vi "GPS Set Target Loop.vi"   [LabVIEW 2009]
uses:
  <vilib>/Platform/TimedLoop/XDataNode/XDataNode.xnode
  <vilib>/Platform/TimedLoop/XDataNode/loadlvalarms.vi
  <vilib>/Platform/TimedLoop/XDataNode/timing_clust.ctl
  <vilib>/Platform/TimedLoop/XDataNode/nitl_modes.ctl
  <vilib>/Platform/TimedLoop/XDataNode/wakeup.ctl
  TypeDefs/State Machine/Main State.ctl
  TypeDefs/Sensor TypeDefs/GPS Data.ctl
  Functional Global Variables/Actions for FG's.ctl
  <vilib>/Platform/TimedLoop/XDataNode/XDNodeRunTimeDep.lvlib
types:
  T1 = typedef "XDNodeRunTimeDep.lvlib/timing_clust.ctl" = cluster{"Expected End [f-1]":u64, "Actual End [f-1]":u64, "Finished Late? [f-1]":bool, "Expected End [i-1]":u64, "Actual End [i-1]":u64, "Finished Late? [i-1]":bool, "Expected Start [i]":u64, "Actual Start [i]":u64, "Expected Start [f]":u64, "Actual Start [f]":u64, "Source Name":string, "Structure Name":string, "Period":i64, "Deadline":i64, "Offset":i64, "Start":i64, "Priority":i32, "Timeout":i32, "Mode":T2, "Wakeup Reason":T3, "Error":errorcluster, "Source Type":string, "Secondary Source Type":string, "Global End Time":u64, "Global Start Time":u64, "Frame Duration":u64, "Iteration Duration":u64, "Assigned CPU":i32, "I/O Scan Engine Mode":u32}
  T2 = typedef "XDNodeRunTimeDep.lvlib/nitl_modes.ctl" = enum32{"No Change", "Process missed periods, maintain original phase", "Discard missed periods, maintain original phase", "Process missed periods, ignore original phase", "Discard missed periods, ignore original phase"}
  T3 = typedef "XDNodeRunTimeDep.lvlib/wakeup.ctl" = enum32{"Normal", "Aborted", "Asynchronous wakeup", "Timing source error", "Timed loop error", "Timeout"}
  T4 = typedef "Main State.ctl" = enum16{"Startup", "Wait for Init", "Initialize Sensors", "Wait for Saftey Disable", "Check Saftey", "Wait for GO", "Run", "Remote Control", "Stop"}
  T5 = typedef "Actions for FG's.ctl" = enum16{"Read", "Write"}
  T6 = typedef "GPS Data.ctl" = cluster{"Latitude":dbl, "Longitude":dbl}
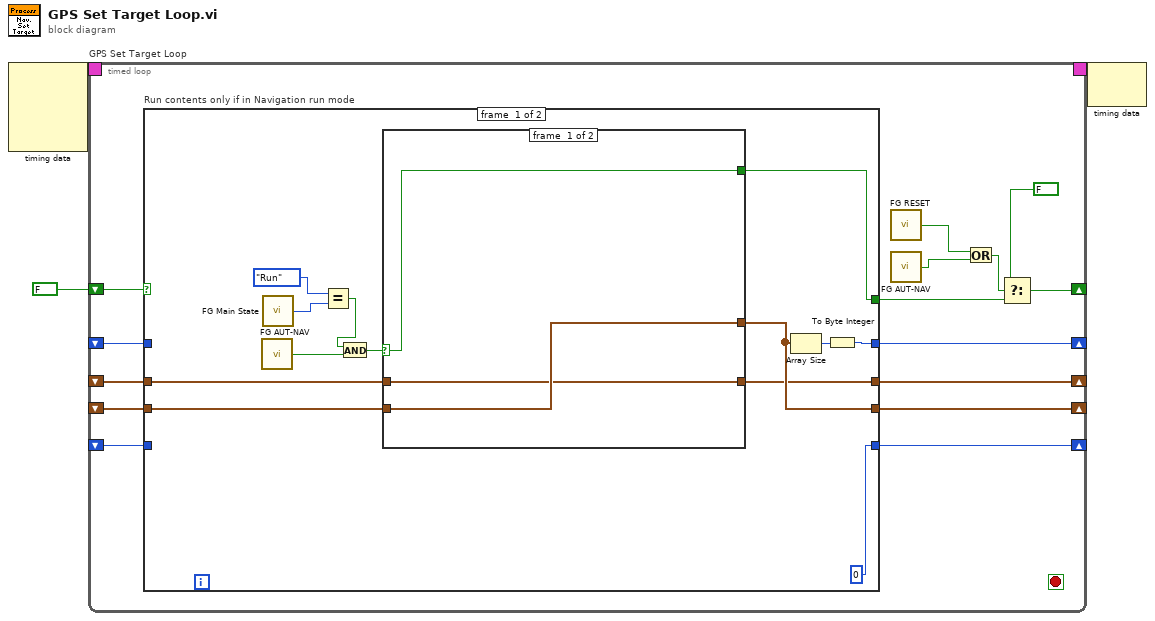
[diagram p0: block diagram]
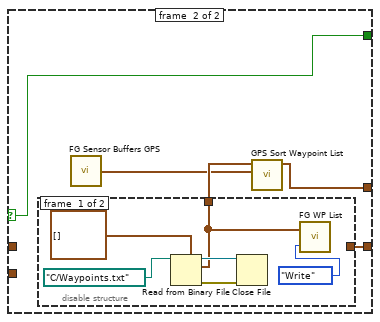
[diagram p2: hidden frame]
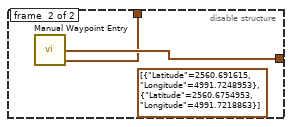
[diagram p3: hidden frame]
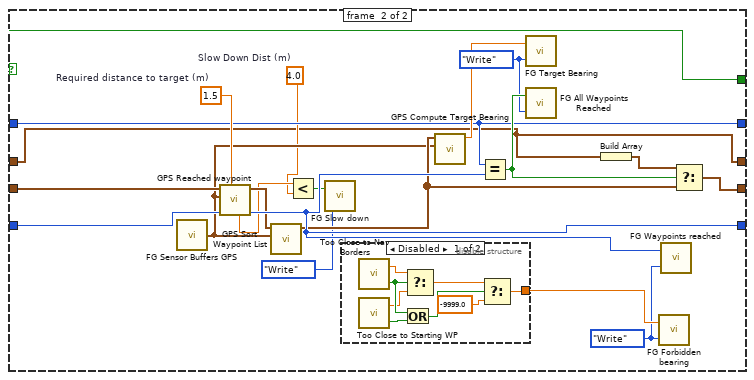
[diagram p4: hidden frame]
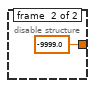
[diagram p5: hidden frame]
diagram:
  n1 = node-c288() -> (w3:T1)  [unwired: 4 in]
  n2 = timed-loop "GPS Set Target Loop" {
    timing: w3 -> [_]
    timing-out: [_] -> w2
    shift-right: [w16] -> _
    shift-left: _ -> [w18]
    shift-right: [w14] -> _
    shift-left: _ -> [w15]
    shift-right: [w10] -> _
    shift-left: FALSE ("t") -> [w9]
    shift-right: [w13] -> _
    shift-left: _ -> [w17]
    shift-right: [w8] -> _
    shift-left: _ -> [w7]
    stop <- _ stop-if-true
    n3 = case "Run contents only if in Navigation run mode" shown="False" w9 {
      selector: w9 -> [_ w57]
      tunnel: w18 -> [_ w67]
      tunnel: w17 -> [_ w56]
      tunnel: [i8 0 ("Number of WP Reached OUT") w66] -> w16
      tunnel: w15 -> [w24 w65]
      tunnel: [w22 w60] -> w14
      tunnel: [w27 w57] -> w11
      tunnel: [w25 w56] -> w13
      tunnel: [w21 w48] -> w8
      tunnel: w7 -> [w20 w48]
      frame #0 {
        n4 = call "FG AUT-NAV.vi"() -> ("Aut/!Nav out"=w19:bool)  [unwired: 2 in]
        n5 = call "FG Main State.vi"() -> ("Main State out"=w28:T4)  [unwired: 2 in]
        n6 = Equal?(x=Main_State."Run" ("Main State out"), y=w28) -> (x = y?=w30:bool)
        n7 = And(x=w30, y=w19) -> (x .and. y?=w31:bool)
        n8 = case shown="True" w31 {
          selector: w31 -> [w34 w39]
          tunnel: [w34 w39] -> w27
          tunnel: w24 -> [w33 _]
          tunnel: [w33 w36] -> w22
          tunnel: [w32 w35] -> w21
          tunnel: w20 -> [w32 _]
          frame #0 {
          }
          frame #1 {
            n9 = disable-structure shown="Enabled" {
              disable-tunnel: [w40 w46] -> w38
              disable-tunnel: [_ w47] -> w35
              frame #0 {
                n10 = Read from Binary File(5:T6[] [] ("Unsorted Waypoint List"), 11:path "C:/Waypoints.txt" ("file path (use dialog)")) -> (0:w44:errorcluster, 2:w40:T6[], 3:w43:refnum<file>)  [unwired: 4 in, 1 out]
                n11 = Close File(refnum=w43, error in=w44) -> ()  [unwired: 2 out]
                n12 = call "FG WP List.vi"("FG Action (Read)"=Actions_for_FG's."Write", "Sorted Waypoints in"=w40) -> ()  [unwired: 1 out]
              }
              frame #1 {
                (unwired) T6[] [{"Latitude"=2560.691615, "Longitude"=4991.7248953}, {"Latitude"=2560.6754953, "Longitude"=4991.7218863}] ("Unsorted Waypoint List")
                n13 = call "Manual Waypoint Entry.vi"() -> ("WP List Out"=w46:T6[], "Nav Course Ending Location"=w47:T6)  [unwired: 3 in, 1 out]
              }
            }
            n14 = call "FG Sensor Buffers GPS.vi"() -> ("GPS Buffer out"=w37:T6)  [unwired: 2 in]
            n15 = call "GPS Sort Waypoint List.vi"("Current co-ordinate"=w37, "Unsorted Waypoint List"=w38) -> ("Sorted Waypoints"=w36:T6[])  [unwired: 9 in]
          }
        }
        n16 = Array Size(array=w22) -> (size(s)=w26:i32)
        n17 = To Byte Integer(number=w26) -> (8bit integer=w25:i8)
      }
      frame #1 {
        w51 = 4.0  # Slow Down Dist (m)
        w58 = Actions_for_FG's."Write" ("FG Action (Read)")
        w63 = Actions_for_FG's."Write" ("FG Action (Read)")
        w62 = 1.5  # Required distance to target (m)
        n18 = call "FG Sensor Buffers GPS.vi"() -> ("GPS Buffer out"=w53:T6)  [unwired: 2 in]
        n19 = call "GPS Reached waypoint.vi"("Required distance to target (meters)"=w62, "Number of WP Reached IN"=w67, "Current Co-ordinates"=w53, "Waypoint List In"=w65) -> ("Number of WP Reached OUT"=w66:i8, "Waypoint List Out"=w55:T6[], "Distance to Target (meters)"=w52:dbl)  [unwired: 4 in, 1 out]
        n20 = call "GPS Sort Waypoint List.vi"("Current co-ordinate"=w53, "Unsorted Waypoint List"=w55) -> ("Sorted Waypoints"=w54:T6[])  [unwired: 9 in]
        n21 = Less?(x=w52, y=w51) -> (x < y?=w50:bool)
        n22 = call "FG Slow down.vi"("FG Action (Read)"=Actions_for_FG's."Write", "Slow down in"=w50) -> ()  [unwired: 1 out]
        n23 = disable-structure shown="Disabled" {
          disable-tunnel: [w69 -9999.0 ("Forbidden bearing in")] -> w64
          frame #0 {
            n24 = call "Too Close to Nav Borders.vi"() -> ("Too Close?"=w73:bool, "Bearing to Avoid"=w72:dbl)  [unwired: 2 in]
            n25 = call "Too Close to Starting WP.vi"() -> ("Too Close?"=w76:bool, "Bearing to Avoid"=w71:dbl)  [unwired: 2 in]
            n26 = Or(x=w73, y=w76) -> (x .or. y?=w75:bool)
            n27 = Select(t=w72, s=w73, f=w71) -> (s? t:f=w70:dbl)
            n28 = Select(t=w70, s=w75, f=-9999.0) -> (s? t:f=w69:dbl)
          }
          frame #1 {
          }
        }
        n29 = call "GPS Compute Target Bearing.vi"("Current co-ordinates"=w53, "GPS Waypoint List Out"=w54) -> ("Target Bearing (degrees)"=w68:dbl)  [unwired: 8 in]
        n30 = Equal?(x=w56, y=w66) -> (x = y?=w59:bool)
        n31 = call "FG Target Bearing.vi"("FG Action (Read)"=w58, "Target Bearing in"=w68) -> ()  [unwired: 1 out]
        n32 = call "FG All Waypoints Reached.vi"("FG Action (Read)"=w58, "All waypoints reached in"=w59) -> ()  [unwired: 1 in, 1 out]
        n33 = Build Array(w48) -> (w61:T6[])
        n34 = call "FG Forbidden bearing.vi"("FG Action (Read)"=w63, "Forbidden bearing in"=w64) -> ()  [unwired: 1 out]
        n35 = call "FG Waypoints reached.vi"("FG Action (Read)"=w63, "Waypoints reached in"=w66) -> ()  [unwired: 1 in, 1 out]
        n36 = Select(t=w61, s=w59, f=w54) -> (s? t:f=w60:T6[])
      }
    }
    n37 = call "FG RESET.vi"() -> ("RESET out"=w6:bool)  [unwired: 2 in]
    n38 = call "FG AUT-NAV.vi"() -> ("Aut/!Nav out"=w5:bool)  [unwired: 2 in]
    n39 = Or(x=w6, y=w5) -> (x .or. y?=w4:bool)
    n40 = Select(t=FALSE, s=w4, f=w11) -> (s? t:f=w10:bool)
  }
  n41 = node-c288(w2) -> ()  [unwired: 1 out]
